vi "Clear GPIB Timeout.vi"(6 "Errors to skip":i32[](array[numeric])=[6, -1073807339, -1073807253, -1073807194, -1073807343, -1073807298, -1073807265], 8 "error in (no error)":errorcluster) -> (0 "error out":errorcluster, 1 "Found listed error":bool, 4 "Original error":errorcluster)   [LabVIEW 2018]
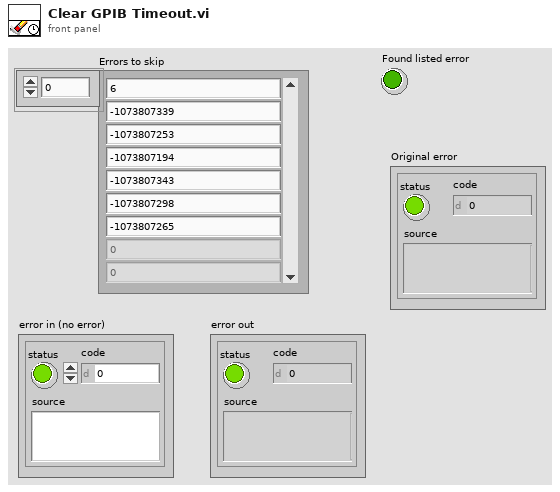
[diagram p1: front panel]
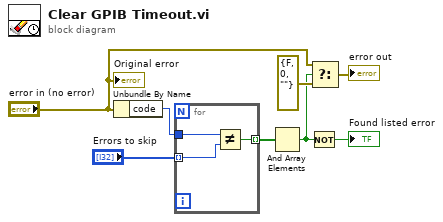
[diagram p0: block diagram]
diagram:
  n1 = Unbundle By Name("error in (no error)") -> ("code"=w8:i32)
  n2 = for {
    tunnel: w8 -> [w9]
    tunnel: [w11] -> w5 mode=indexing
    tunnel: "Errors to skip" -> [w10] mode=indexing
    n3 = Not Equal?(x=w9, y=w10) -> (x != y?=w11:bool)
  }
  n4 = And Array Elements(Boolean array=w5) -> (logical AND=w3:bool)
  n5 = Not(x=w3) -> (.not. x?=→"Found listed error":bool)
  n6 = Select(t="error in (no error)", s=w3, f=errorcluster {"status"=FALSE, "code"=0, "source"=""} ("error out")) -> (s? t:f=→"error out":errorcluster)
  "Original error" <- "error in (no error)"
